vi "Switch_FindCOM.vi"(2 "error in (no error)":errorcluster) -> (0 "错误输出":errorcluster, 1 "VISA resource out":refnum<visa-resource-name>)   [LabVIEW 2018, in "Switch.lvlib"]
uses:
  Switch.lvlib
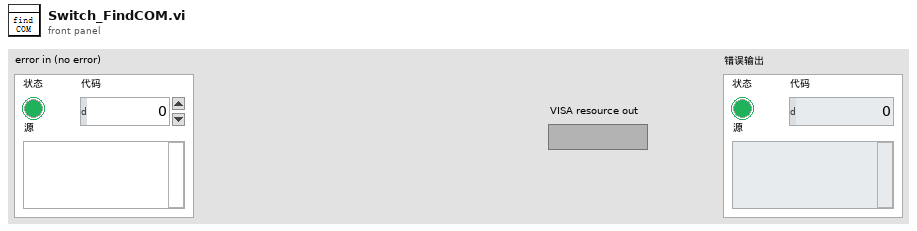
[diagram p1: front panel]
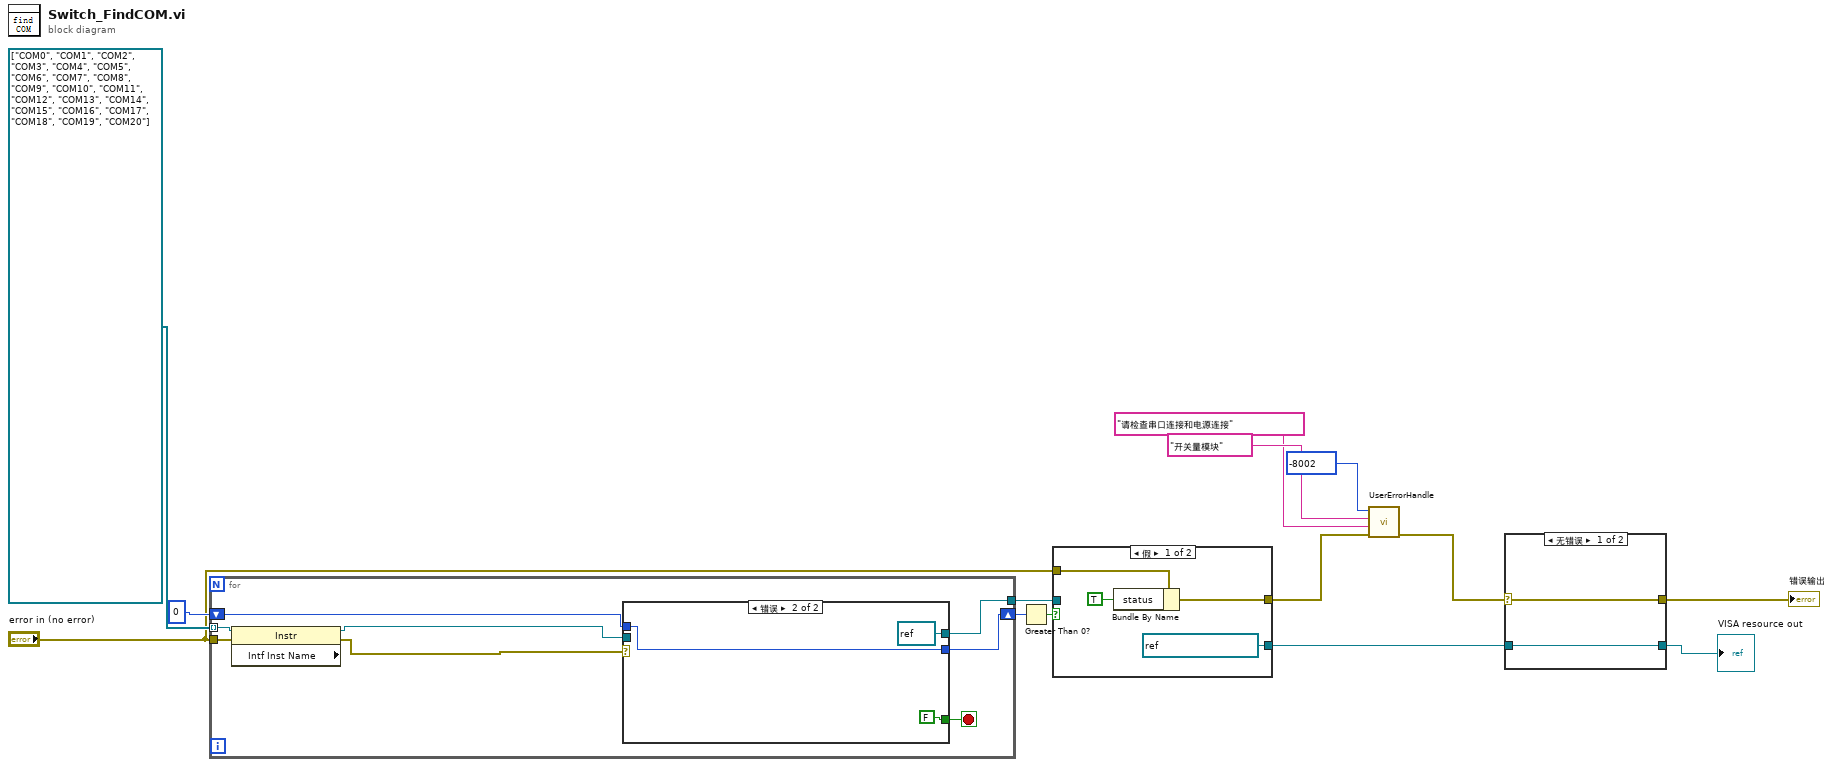
[diagram p0: block diagram]
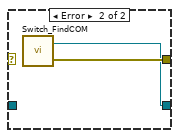
[diagram p2: hidden frame]
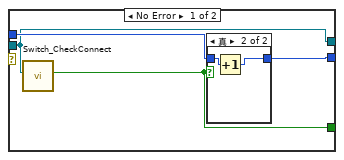
[diagram p4: hidden frame]
diagram:
  n1 = for {
    tunnel: refnum<visa-resource-name>[] ["COM0", "COM1", "COM2", "COM3", "COM4", "COM5", "COM6", "COM7", "COM8", "COM9", "COM10", "COM11", "COM12", "COM13", "COM14", "COM15", "COM16", "COM17", "COM18", "COM19", "COM20"] ("添加的数组") -> [w21] mode=indexing
    tunnel: "error in (no error)" -> [w22]
    shift-right: [w18] -> w12
    shift-left: 0 -> [w19]
    tunnel: [w16] -> w10
    stop <- w17 stop-if-true
    n2 = property class="Instr" props=["Intf Inst Name"](reference=w21, error in=w22) -> (reference out=w20:refnum<visa-resource-name>, error out=w15:errorcluster)  [unwired: 1 out]
    n3 = case shown="错误" w15 {
      tunnel: w20 -> [w23 _]
      tunnel: w19 -> [w26 w31]
      tunnel: [w25 w31] -> w18
      tunnel: [w24 FALSE] -> w17
      tunnel: [w23 refnum<visa-resource-name> refnum ("VISA resource name")] -> w16
      frame No Error {
        n4 = call "Switch_CheckConnect.vi"("COM"=w23) -> ("通信成功？"=w24:bool)  [unwired: 10 in]
        n5 = case shown="真" w24 {
          tunnel: w26 -> [w27 w29]
          tunnel: [w27 w28] -> w25
          frame False {
          }
          frame True {
            n6 = Increment(x=w29) -> (x+1=w28:i32)
          }
        }
      }
      frame Error {
      }
    }
  }
  n7 = Greater Than 0?(x=w12) -> (x > 0?=w11:bool)
  n8 = case shown="假" w11 {
    tunnel: "error in (no error)" -> [w36 w37]
    tunnel: [w34 w37] -> w6
    tunnel: [refnum<visa-resource-name> refnum ("VISA resource name") w38] -> w2
    tunnel: w10 -> [_ w38]
    frame False {
      n9 = Bundle By Name(cluster=w36, "status"=TRUE) -> (w34:errorcluster)
    }
    frame True {
    }
  }
  n10 = call "UserErrorHandle.vi"("错误输入"=w6, "错误解释"="请检查串口连接和电源连接", "错误源"="开关量模块", "错误编号"=-8002) -> ("错误输出"=w5:errorcluster)  [unwired: 7 in]
  n11 = case shown="无错误" w5 {
    selector: w5 -> [w40 _]
    tunnel: [w40 w42] -> w4
    tunnel: [w39 w41] -> w3
    tunnel: w2 -> [w39 _]
    frame No Error {
    }
    frame Error {
      n12 = call "Switch_FindCOM.vi"() -> ("错误输出"=w42:errorcluster, "VISA resource out"=w41:refnum<visa-resource-name>)  [unwired: 2 in]
    }
  }
  "VISA resource out" <- w3
  "错误输出" <- w4
